vi "Calculate IM Freqs.vi"(6 "Low-side?":bool, 8 "F2 (Carrier 2)":dbl, 9 "F1 (Carrier 1)":dbl, 10 "SingleIM? (f)":bool, 11 "BaseOrder":u8) -> (3 "IM Frequencies":dbl[](array[numeric]))   [LabVIEW 2011]
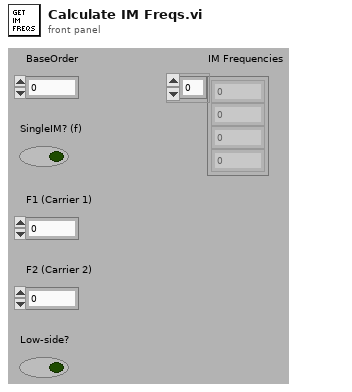
[diagram p1: front panel]
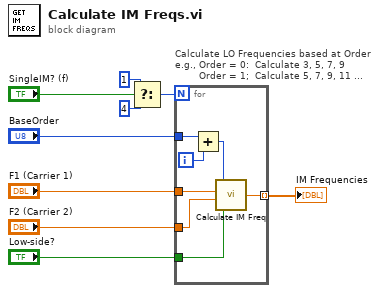
[diagram p0: block diagram]
diagram:
  n1 = Select(t=1, s="SingleIM? (f)", f=4) -> (s? t:f=w6:i32)
  n2 = for "Calculate LO Frequencies based at Order\ne.g., Order = 0:  Calculate 3, 5, 7, 9\n        Order = 1;  Calculate 5, 7, 9, 11 ..." {
    N: w6 -> [_]
    tunnel: "F1 (Carrier 1)" -> [w16]
    tunnel: "F2 (Carrier 2)" -> [w14]
    tunnel: "BaseOrder" -> [w12]
    tunnel: [w15] -> w9 mode=indexing
    tunnel: "Low-side?" -> [w13]
    i -> [w11]
    n3 = Add(x=w12, y=w11) -> (x+y=w10:i32)
    n4 = call "Calculate IM Freq.vi"("Low-side?"=w13, "F2 (Carrier 2)"=w14, "F1 (Carrier 1)"=w16, "BaseImOrder"=w10) -> ("IM Frequency"=w15:dbl)
  }
  "IM Frequencies" <- w9
